vi "Dateien_updaten.vi"(8 "Fehler in":errorcluster, 11 "Cluster in":T1={"Initialisierung"={"Online?"=FALSE, "Grundpfad"=path "", "Kamera Oben"="", "IP-Adresse Flüssiglinse"="", "Flüssiglinse"=refnum, "Kamera Unten"="", "IP-Adresse SPS"="", "SPS-Verbindung"={"TCP Connection Ref"=refnum, "IP address"="", "timeout ms"=5000, "Connected?"=FALSE, "PLC Type"=enum."S7 1200", "Rack S7 400"=0, "Slot S7 400"=0, "PDU Size"=0, "connection semaphore"=refnum}, "IP-Adresse Lichtgitter"="", "Lichtgitter"=refnum, "Skalierungsfaktor"=0.0, "Bilder Oben"=[], "Bild Unten"=refnum, "Bild Ausschnitt Unten"=refnum}, "Einstellungen"={"Gesamtablauf gestartet"=FALSE, "i. O. Bilder speichern"=FALSE, "Bildspeicherung Offline"=FALSE, "Ausgewähltes Offline-Datum"="", "Ausgewähltes Offline-Teil"="", "Speicherpfad Bilder"=path ""}, "Artikeldaten"={"Artikelnummer"="", "Fertigungsauftrag"="", "Muster ISO"=refnum, "Belichtungszeit Referenzmarken"=0.0, "Fokus Referenzmarken"=0.0, "Belichtungszeit ISO"=0.0, "Fokus ISO"=0.0, "Belichtungszeit Unten"=0.0, "Kontaktanzahl"=0, "Aktueller Kontakt"=0, "Kontaktposition"={"x"=0.0, "y"=0.0}, "ISO-Muster nicht vorhanden"=FALSE, "Winkel ISO"=0.0, "Mittelpunkt ISO"={"x"=0.0, "y"=0.0}}, "Werte Kamera Oben"={"Koordinatensystem"={"Punkt x-Achse"={"X"=0.0, "Y"=0.0}, "Ursprung"={"X"=0.0, "Y"=0.0}, "Punkt y-Achse"={"X"=0.0, "Y"=0.0}}, "Position Kontakt"={"x"=0.0, "y"=0.0}, "Durchmesser Loch"=0.0, "Winkel Kontakt"=0.0}, "Werte Kamera Unten"={"Prüfung Unten n. i. O."=FALSE}, "Werte Lichtgitter"={"Messwerte Referenzmarken"=[], "Mittelpunkt Referenzmarken"={"x"=0.0, "y"=0.0}, "Messwerte Kontakt"=[], "Offset"={"x"=0.0, "y"=0.0}}, "Rückmeldungen"={"Koordinaten ermittelt"=FALSE, "Vermessung Lichtgitter fertig"=FALSE, "Nachkontrolle Kamera Unten fertig"=FALSE}, "Fehler"={"Referenzen nicht gefunden"=FALSE, "Kontakt nicht gefunden"=FALSE, "Referenzen nicht in Lichtgitter"=FALSE, "Kontakt zu groß"=FALSE, "Kontakt zu klein"=FALSE}, "Statistik"={"Statistiken"=[]}, "Timer"={"Timer Start Position"=0, "Timer Start Lichtgitter"=0, "Timer Start Kamera Unten"=0}}) -> (0 "Fehler out":errorcluster, 3 "Cluster out":T1={"Initialisierung"={"Online?"=FALSE, "Grundpfad"=path "", "Kamera Oben"="", "IP-Adresse Flüssiglinse"="", "Flüssiglinse"=refnum, "Kamera Unten"="", "IP-Adresse SPS"="", "SPS-Verbindung"={"TCP Connection Ref"=refnum, "IP address"="", "timeout ms"=5000, "Connected?"=FALSE, "PLC Type"=enum."S7 1200", "Rack S7 400"=0, "Slot S7 400"=0, "PDU Size"=0, "connection semaphore"=refnum}, "IP-Adresse Lichtgitter"="", "Lichtgitter"=refnum, "Skalierungsfaktor"=0.0, "Bilder Oben"=[], "Bild Unten"=refnum, "Bild Ausschnitt Unten"=refnum}, "Einstellungen"={"Gesamtablauf gestartet"=FALSE, "i. O. Bilder speichern"=FALSE, "Bildspeicherung Offline"=FALSE, "Ausgewähltes Offline-Datum"="", "Ausgewähltes Offline-Teil"="", "Speicherpfad Bilder"=path ""}, "Artikeldaten"={"Artikelnummer"="", "Fertigungsauftrag"="", "Muster ISO"=refnum, "Belichtungszeit Referenzmarken"=0.0, "Fokus Referenzmarken"=0.0, "Belichtungszeit ISO"=0.0, "Fokus ISO"=0.0, "Belichtungszeit Unten"=0.0, "Kontaktanzahl"=0, "Aktueller Kontakt"=0, "Kontaktposition"={"x"=0.0, "y"=0.0}, "ISO-Muster nicht vorhanden"=FALSE, "Winkel ISO"=0.0, "Mittelpunkt ISO"={"x"=0.0, "y"=0.0}}, "Werte Kamera Oben"={"Koordinatensystem"={"Punkt x-Achse"={"X"=0.0, "Y"=0.0}, "Ursprung"={"X"=0.0, "Y"=0.0}, "Punkt y-Achse"={"X"=0.0, "Y"=0.0}}, "Position Kontakt"={"x"=0.0, "y"=0.0}, "Durchmesser Loch"=0.0, "Winkel Kontakt"=0.0}, "Werte Kamera Unten"={"Prüfung Unten n. i. O."=FALSE}, "Werte Lichtgitter"={"Messwerte Referenzmarken"=[], "Mittelpunkt Referenzmarken"={"x"=0.0, "y"=0.0}, "Messwerte Kontakt"=[], "Offset"={"x"=0.0, "y"=0.0}}, "Rückmeldungen"={"Koordinaten ermittelt"=FALSE, "Vermessung Lichtgitter fertig"=FALSE, "Nachkontrolle Kamera Unten fertig"=FALSE}, "Fehler"={"Referenzen nicht gefunden"=FALSE, "Kontakt nicht gefunden"=FALSE, "Referenzen nicht in Lichtgitter"=FALSE, "Kontakt zu groß"=FALSE, "Kontakt zu klein"=FALSE}, "Statistik"={"Statistiken"=[]}, "Timer"={"Timer Start Position"=0, "Timer Start Lichtgitter"=0, "Timer Start Kamera Unten"=0}})   [LabVIEW 2024]
doc: "Speichert die Statistiken und die Kontaktnummer in die jeweiligen Dateien."
uses:
  Typdefinitionen/Cluster.ctl
  <vilib>/userDefined/High Color/IMAQdx.ctl
  <vilib>/DATA AHEAD/SP7/typedefs/S7 Connection.ctl
  <vilib>/DATA AHEAD/SP7/typedefs/PLC Type.ctl
  <vilib>/vision/Image Controls.llb/IMAQ Image.ctl
  Typdefinitionen/Koordinatensystem.ctl
  Typdefinitionen/Statistik.ctl
  <vilib>/Utility/config.llb/Write Key (U32).vi
  <vilib>/Utility/config.llb/NI_LVConfig.lvlib
  <vilib>/Utility/config.llb/Write Key (Double).vi
  <vilib>/DATA AHEAD/SP7/SP7.lvlib
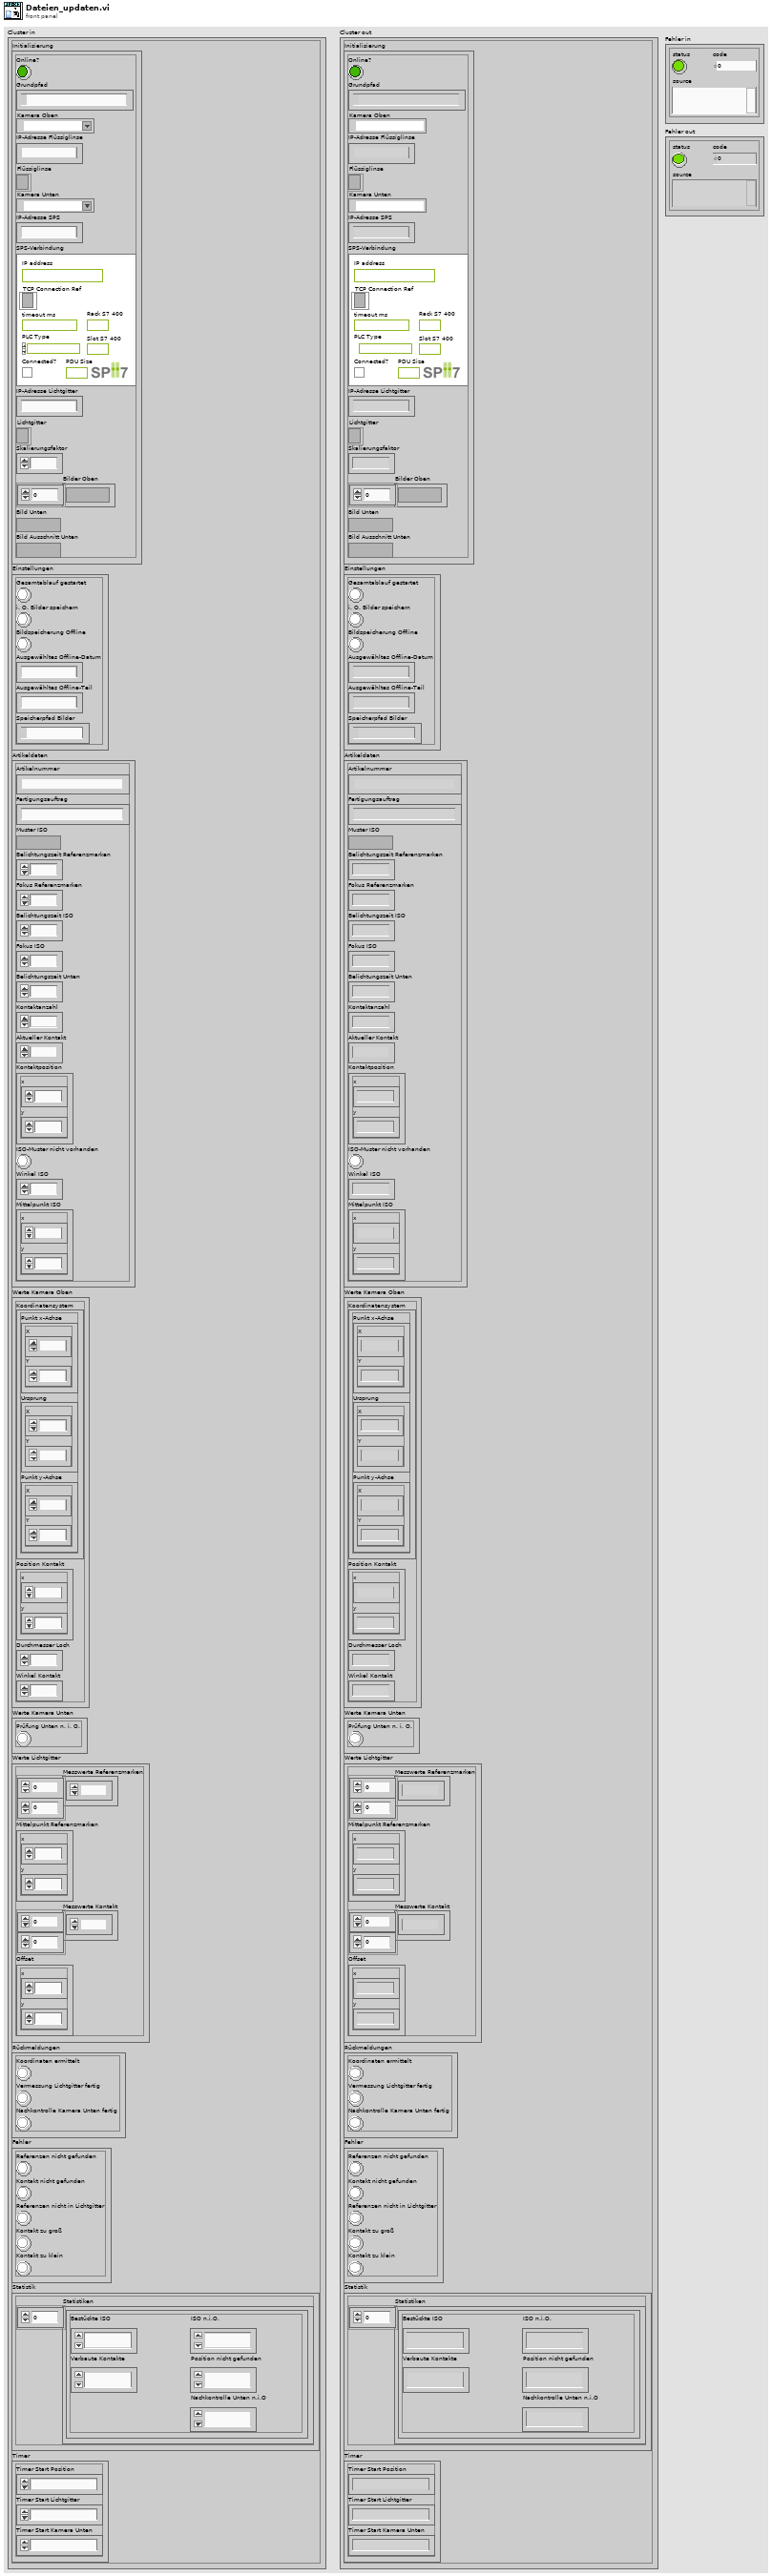
[diagram p1: front panel]
types:
  T1 = typedef "Cluster.ctl" = cluster{"Initialisierung":cluster{"Online?":bool, "Grundpfad":path, "Kamera Oben":T2, "IP-Adresse Flüssiglinse":string, "Flüssiglinse":refnum<k5>, "Kamera Unten":T2, "IP-Adresse SPS":string, "SPS-Verbindung":T3, "IP-Adresse Lichtgitter":string, "Lichtgitter":refnum<k5>, "Skalierungsfaktor":dbl, "Bilder Oben":T6[], "Bild Unten":T6, "Bild Ausschnitt Unten":T6}, "Einstellungen":cluster{"Gesamtablauf gestartet":bool, "i. O. Bilder speichern":bool, "Bildspeicherung Offline":bool, "Ausgewähltes Offline-Datum":string, "Ausgewähltes Offline-Teil":string, "Speicherpfad Bilder":path}, "Artikeldaten":cluster{"Artikelnummer":string, "Fertigungsauftrag":string, "Muster ISO":T6, "Belichtungszeit Referenzmarken":dbl, "Fokus Referenzmarken":dbl, "Belichtungszeit ISO":dbl, "Fokus ISO":dbl, "Belichtungszeit Unten":dbl, "Kontaktanzahl":u32, "Aktueller Kontakt":i16, "Kontaktposition":cluster{"x":sgl, "y":sgl}, "ISO-Muster nicht vorhanden":bool, "Winkel ISO":sgl, "Mittelpunkt ISO":cluster{"x":dbl, "y":dbl}}, "Werte Kamera Oben":cluster{"Koordinatensystem":T7, "Position Kontakt":cluster{"x":dbl, "y":dbl}, "Durchmesser Loch":dbl, "Winkel Kontakt":dbl}, "Werte Kamera Unten":cluster{"Prüfung Unten n. i. O.":bool}, "Werte Lichtgitter":cluster{"Messwerte Referenzmarken":dbl[][], "Mittelpunkt Referenzmarken":cluster{"x":dbl, "y":dbl}, "Messwerte Kontakt":dbl[][], "Offset":cluster{"x":dbl, "y":dbl}}, "Rückmeldungen":cluster{"Koordinaten ermittelt":bool, "Vermessung Lichtgitter fertig":bool, "Nachkontrolle Kamera Unten fertig":bool}, "Fehler":cluster{"Referenzen nicht gefunden":bool, "Kontakt nicht gefunden":bool, "Referenzen nicht in Lichtgitter":bool, "Kontakt zu groß":bool, "Kontakt zu klein":bool}, "Statistik":cluster{"Statistiken":T8[]}, "Timer":cluster{"Timer Start Position":u32, "Timer Start Lichtgitter":u32, "Timer Start Kamera Unten":u32}}
  T2 = typedef "IMAQdx.ctl" = refnum<k21>
  T3 = typedef "SP7.lvlib/S7 Connection.ctl" = cluster{"TCP Connection Ref":refnum<k5>, "IP address":string, "timeout ms":i32, "Connected?":bool, "PLC Type":T4, "Rack S7 400":u8, "Slot S7 400":u8, "PDU Size":u16, "connection semaphore":T5}
  T4 = typedef "SP7.lvlib/PLC Type.ctl" = enum16{"S7 200", "S7 300/400", "S7 1200", "S7 1500", "LOGO!8"}
  T5 = typedef "Semaphore RefNum" = refnum<k1>
  T6 = typedef "IMAQ Image.ctl" = refnum<image>
  T7 = typedef "Koordinatensystem.ctl" = cluster{"Punkt x-Achse":cluster{"X":sgl, "Y":sgl}, "Ursprung":cluster{"X":sgl, "Y":sgl}, "Punkt y-Achse":cluster{"X":sgl, "Y":sgl}}
  T8 = typedef "Statistik.ctl" = cluster{"Bestückte ISO":u32, "Verbaute Kontakte":u32, "ISO n.i.O.":u32, "Nachkontrolle Unten n.i.O":u32, "Position nicht gefunden":u32}
  T9 = typedef "NI_LVConfig.lvlib/Config Data RefNum.ctl" = refnum<k1>
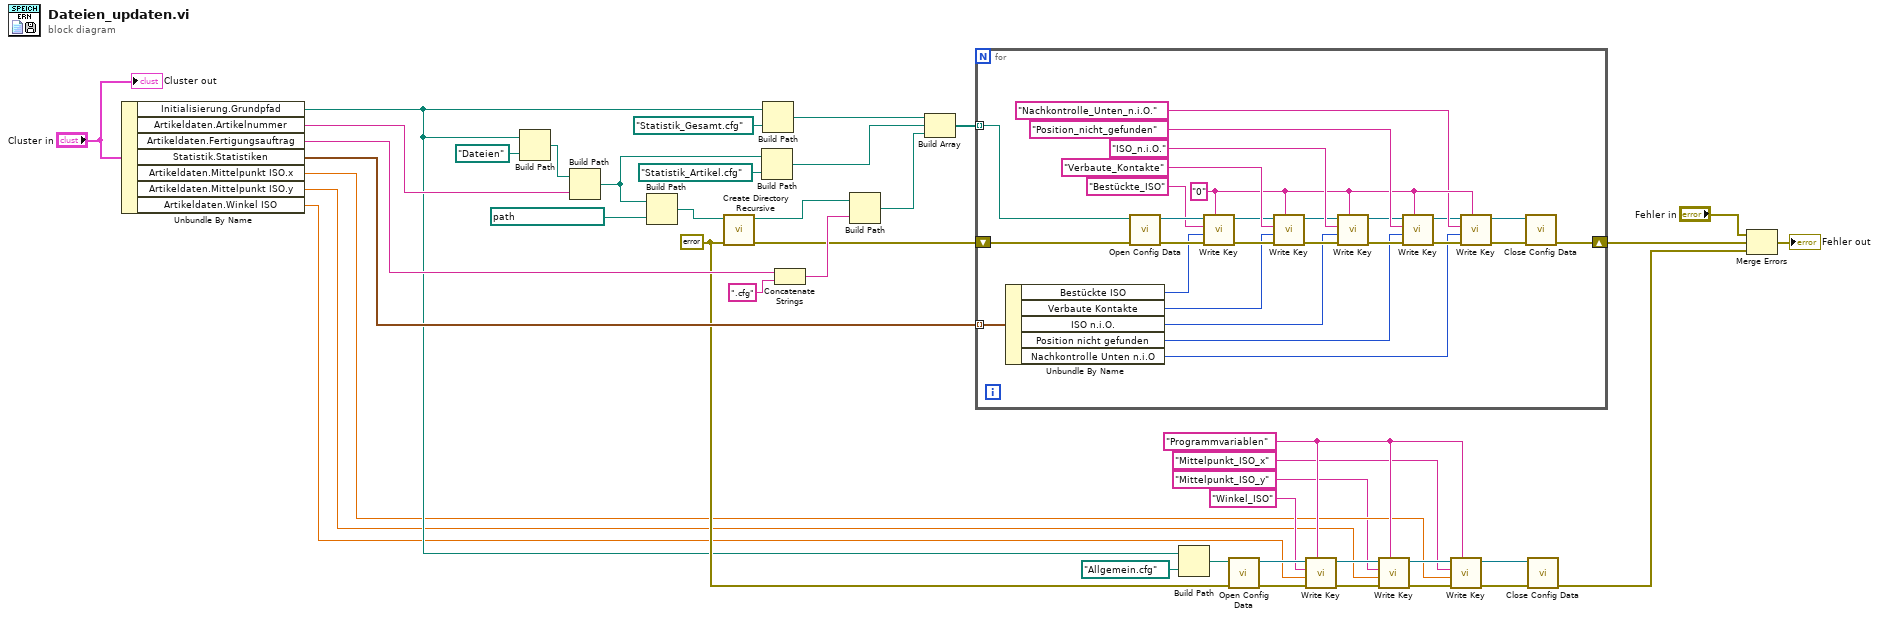
[diagram p0: block diagram]
diagram:
  w5 = "Programmvariablen" ("section")
  w16 = errorcluster {"status"=FALSE, "code"=0, "source"=""} ("error in (no error)")
  n1 = Unbundle By Name("Cluster in") -> ("Initialisierung.Grundpfad"=w13:path, "Artikeldaten.Artikelnummer"=w36:string, "Artikeldaten.Fertigungsauftrag"=w27:string, "Statistik.Statistiken"=w39:T8[], "Artikeldaten.Mittelpunkt ISO.x"=w3:dbl, "Artikeldaten.Mittelpunkt ISO.y"=w4:dbl, "Artikeldaten.Winkel ISO"=w7:sgl)
  n2 = Build Path(base path=w13, name or relative path=path "Dateien") -> (appended path=w37:path)
  n3 = Build Path(base path=w37, name or relative path=w36) -> (appended path=w32:path)
  n4 = Build Path(base path=w32, name or relative path=path "Fertigungsaufträge") -> (appended path=w24:path)
  n5 = call <vilib>:"Create Directory Recursive.vi"("error in (no error)"=w16, "directory"=w24) -> ("error out"=w22:errorcluster, "directory copy"=w23:path)  [unwired: 3 in, 1 out]
  n6 = Build Path(base path=w32, name or relative path=path "Statistik_Artikel.cfg") -> (appended path=w30:path)
  n7 = Build Path(base path=w13, name or relative path=path "Statistik_Gesamt.cfg") -> (appended path=w33:path)
  n8 = Concatenate Strings(w27, ".cfg" ("string")) -> (w25:string)
  n9 = Build Path(base path=w23, name or relative path=w25) -> (appended path=w29:path)
  n10 = Build Array(w33, w30, w29) -> (w28:path[])
  n11 = for {
    shift-right: [w51] -> w14
    shift-left: w22 -> [w50]
    tunnel: w39 -> [w49] mode=indexing
    tunnel: w28 -> [w43] mode=indexing
    w59 = "0" ("section")
    n12 = Unbundle By Name(w49) -> ("Bestückte ISO"=w48:u32, "Verbaute Kontakte"=w47:u32, "ISO n.i.O."=w46:u32, "Position nicht gefunden"=w45:u32, "Nachkontrolle Unten n.i.O"=w44:u32)
    n13 = call <vilib>:"Open Config Data.vi"("error in (no error)"=w50, "configuration file path"=w43) -> ("error out"=w66:errorcluster, "refnum"=w69:T9)  [unwired: 7 in, 1 out]
    n14 = call-poly <vilib>:"Write Key.vi"("section"=w59, "error in (no error)"=w66, "value"=w48, "key"="Bestückte_ISO", "refnum"=w69) -> ("error out"=w67:errorcluster, "refnum out"=w52:T9)  [unwired: 4 in, 1 out]
    n15 = call-poly <vilib>:"Write Key.vi"("section"=w59, "error in (no error)"=w67, "value"=w47, "key"="Verbaute_Kontakte", "refnum"=w52) -> ("error out"=w65:errorcluster, "refnum out"=w53:T9)  [unwired: 4 in, 1 out]
    n16 = call-poly <vilib>:"Write Key.vi"("section"=w59, "error in (no error)"=w65, "value"=w46, "key"="ISO_n.i.O.", "refnum"=w53) -> ("error out"=w64:errorcluster, "refnum out"=w54:T9)  [unwired: 4 in, 1 out]
    n17 = call-poly <vilib>:"Write Key.vi"("section"=w59, "error in (no error)"=w64, "value"=w45, "key"="Position_nicht_gefunden", "refnum"=w54) -> ("error out"=w63:errorcluster, "refnum out"=w55:T9)  [unwired: 4 in, 1 out]
    n18 = call-poly <vilib>:"Write Key.vi"("section"=w59, "error in (no error)"=w63, "value"=w44, "key"="Nachkontrolle_Unten_n.i.O.", "refnum"=w55) -> ("error out"=w57:errorcluster, "refnum out"=w56:T9)  [unwired: 4 in, 1 out]
    n19 = call <vilib>:"Close Config Data.vi"("error in (no error)"=w57, "refnum"=w56) -> ("error out"=w51:errorcluster)  [unwired: 8 in, 1 out]
  }
  n20 = Build Path(base path=w13, name or relative path=path "Allgemein.cfg") -> (appended path=w20:path)
  n21 = call <vilib>:"Open Config Data.vi"("error in (no error)"=w16, "configuration file path"=w20) -> ("error out"=w19:errorcluster, "refnum"=w18:T9)  [unwired: 7 in, 1 out]
  n22 = call-poly <vilib>:"Write Key.vi"("section"=w5, "error in (no error)"=w19, "value"=w7, "key"="Winkel_ISO", "refnum"=w18) -> ("error out"=w10:errorcluster, "refnum out"=w12:T9)  [unwired: 4 in, 1 out]
  n23 = call-poly <vilib>:"Write Key.vi"("section"=w5, "error in (no error)"=w10, "value"=w4, "key"="Mittelpunkt_ISO_y", "refnum"=w12) -> ("error out"=w8:errorcluster, "refnum out"=w6:T9)  [unwired: 4 in, 1 out]
  n24 = call-poly <vilib>:"Write Key.vi"("section"=w5, "error in (no error)"=w8, "value"=w3, "key"="Mittelpunkt_ISO_x", "refnum"=w6) -> ("error out"=w9:errorcluster, "refnum out"=w11:T9)  [unwired: 4 in, 1 out]
  n25 = call <vilib>:"Close Config Data.vi"("error in (no error)"=w9, "refnum"=w11) -> ("error out"=w15:errorcluster)  [unwired: 8 in, 1 out]
  n26 = Merge Errors("Fehler in", w14, w15) -> (→"Fehler out":errorcluster)
  "Cluster out" <- "Cluster in"
